vi "GenerateChangedLibrariesList.vi"(6 "GUI Mode? {F)":bool, 8 "error in (no error)":errorcluster) -> (0 "error out":errorcluster)   [LabVIEW 2023, in "CICD.lvlib"]
uses:
  CICD.lvlib
  ead0c1dc-4abe-4fdf-93af-0a2c3e7fff4b.vi
  <vilib>/Wiresmith Technology/G CLI/CLI Class/CLI.lvclass
panel:
  in  "Tab Control":enum32{"GUI Mode", "CLI Mode"}(tab)=enum."CLI Mode"
  in  "Workspace Path":path=path "E:/sw-deps-monitor"
  out "Args":string[](array[string])=["E:\\sw-deps-monitor"]
  # "When in GUI Mode, the controls will be used, \nin CLI Mode the Args will be used"
  # "Command to run the VI from terminal\n\ng-cli -v --lv-ver 2023 --arch 32 \"E:\\sw-deps-monitor\\CICD\\CheckModifiedVIs\\GenerateChangedLibrariesList.vi\" -- \"E:\\sw-deps-monitor\""
  # "Workspace Path"
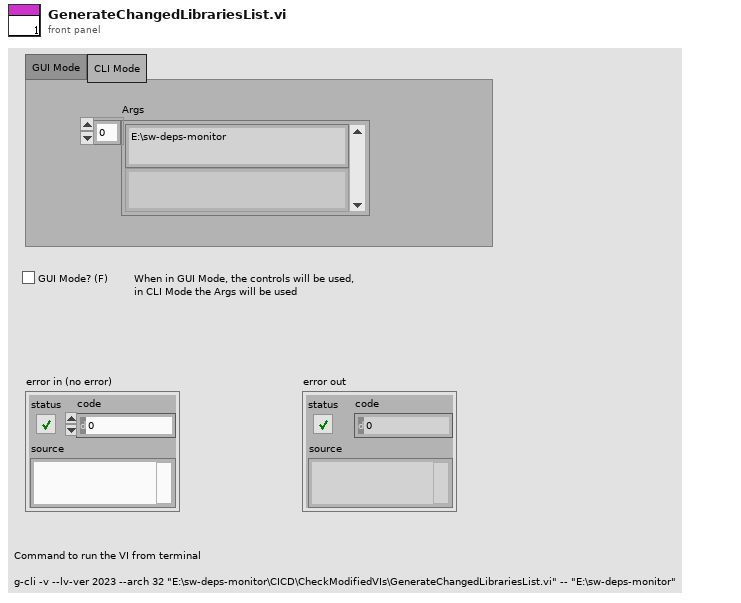
[diagram p1: front panel]
types:
  T1 = enum16{"open", "replace", "create", "open or create", "replace or create", "replace or create with confirmation"}
  T2 = typedef "CICD.lvlib/CICDPathConfigs.ctl" = cluster{"GlobalIncludePaths":path[], "GlobalExcludePaths":path[], "BuildSpecsIncludePaths":path[], "ActualDepsIncludePaths":path[], "WorkspacePath":path, "SourceFolderPaths":path[], "ChangedFilesLogpaths":map{string, path}}
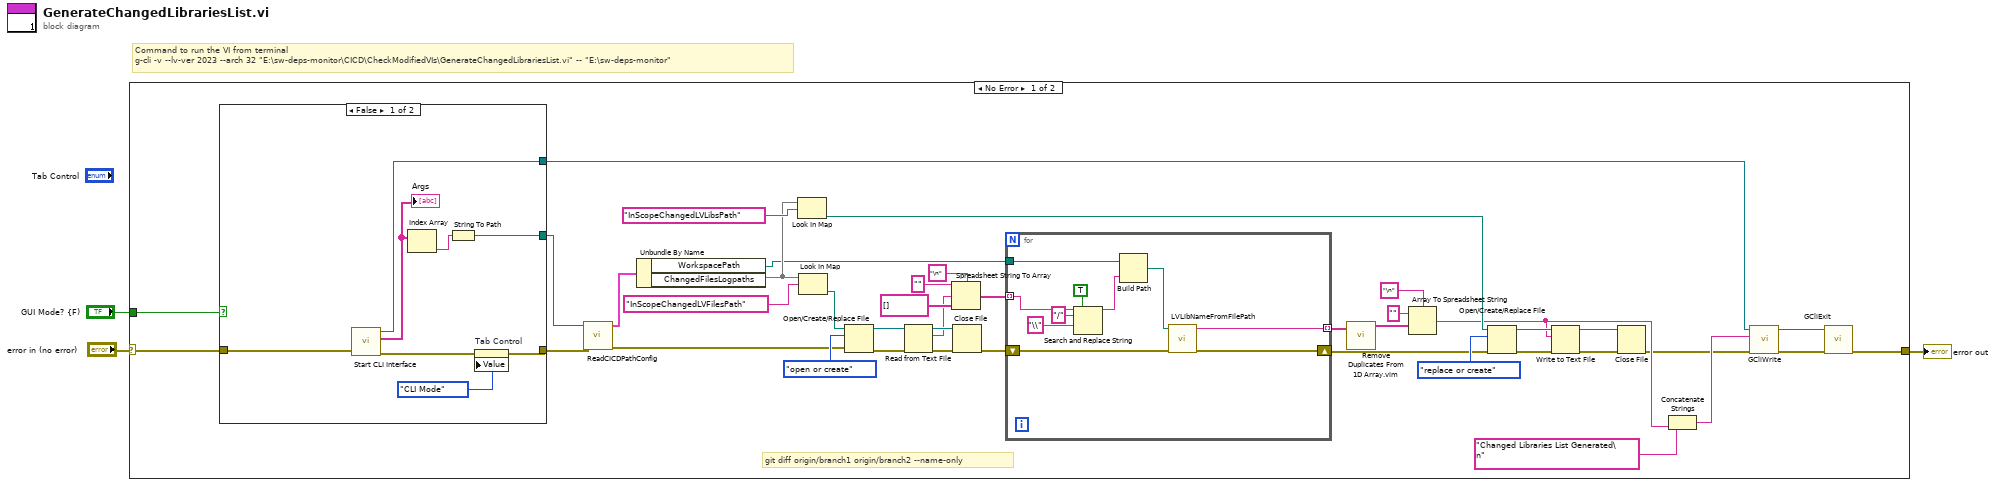
[diagram p0: block diagram]
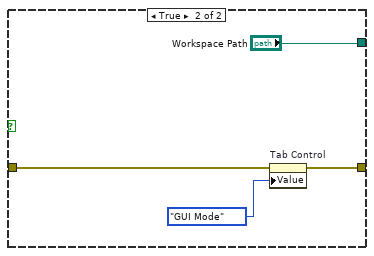
[diagram p2: hidden frame]
diagram:
  # "Command to run the VI from terminal\ng-cli -v --lv-ver 2023 --arch 32 \"E:\\sw-deps-monitor\\CICD\\CheckModifiedVIs\\GenerateChangedLibrariesList.vi\" -- \"E:\\sw-deps-monitor\""
  n1 = case shown="No Error" "error in (no error)" {
    selector: "error in (no error)" -> [w43 w67]
    tunnel: "GUI Mode? {F)" -> [w44 _]
    tunnel: [w39 w67] -> w1
    frame No Error {
      # "git diff origin/branch1 origin/branch2 --name-only"
      n2 = case shown="False" w44 {
        tunnel: [w61 "Workspace Path"] -> w35
        tunnel: w43 -> [w60 w65]
        tunnel: [w58 w63] -> w34
        tunnel: [w59 _] -> w41
        frame False {
          n3 = call <vilib>:"Start CLI Interface.vi"("error in (no error)"=w60) -> ("error out"=w56:errorcluster, "Custom Parameters"=w55:string[], "CLI out"=w59:refnum<class "CLI.lvclass">)  [unwired: 7 in, 1 out]
          "Args" <- w55
          n4 = Index Array(array=w55) -> (element=w62:string)  [unwired: 1 in]
          n5 = String To Path(string=w62) -> (path=w61:path)
          n6 = property on="Tab Control" class="TabCtl (strict)"(error in=w56, "Value"=enum32{"GUI Mode", "CLI Mode"}."CLI Mode" ("Tab Control")) -> (error out=w58:errorcluster)  [unwired: 1 in, 1 out]
        }
        frame True {
          n7 = property on="Tab Control" class="TabCtl (strict)"(error in=w65, "Value"=enum32{"GUI Mode", "CLI Mode"}."GUI Mode" ("Tab Control")) -> (error out=w63:errorcluster)  [unwired: 1 in, 1 out]
        }
      }
      n8 = call "ReadCICDPathConfig.vi"("error in (no error)"=w34, "Workspace Path"=w35) -> ("error out"=w23:errorcluster, "CICD Path Config Out"=w33:T2)  [unwired: 8 in]
      n9 = Unbundle By Name(w33) -> ("WorkspacePath"=w13:path, "ChangedFilesLogpaths"=w21:map{string, path})
      n10 = Look In Map(map=w21, key="InScopeChangedLVLibsPath") -> (value=w20:path)  [unwired: 1 in, 1 out]
      n11 = Look In Map(map=w21, key="InScopeChangedLVFilesPath") -> (value=w31:path)  [unwired: 1 in, 1 out]
      n12 = Open/Create/Replace File(file path (use dialog)=w31, error in=w23, operation (0:open)=T1."open or create") -> (refnum out=w30:refnum<file>, error out=w29:errorcluster)  [unwired: 3 in, 1 out]
      n13 = Read from Text File(file (use dialog)=w30, error in=w29) -> (refnum out=w28:refnum<file>, text=w25:string, error out=w27:errorcluster)  [unwired: 2 in, 1 out]
      n14 = Spreadsheet String To Array(delimiter (Tab)="\n", format string="", spreadsheet string=w25, array type (2D Dbl)=string[] []) -> (array=w14:string[])
      n15 = Close File(refnum=w28, error in=w27) -> (error out=w12:errorcluster)  [unwired: 1 out]
      n16 = for {
        tunnel: w14 -> [w49] mode=indexing
        tunnel: w13 -> [w54]
        tunnel: [w51] -> w5 mode=indexing
        shift-right: [w50] -> w9
        shift-left: w12 -> [w53]
        n17 = Search and Replace String(replace all?=TRUE ("replace all? (F)"), input string=w49, search string="/", replace string="\\" ("replace string (\"\")")) -> (result string=w45:string)  [unwired: 4 in, 3 out]
        n18 = Build Path(base path=w54, name or relative path=w45) -> (appended path=w52:path)
        n19 = call "LVLibNameFromFilePath.vi"("error in (no error)"=w53, "LV File Path"=w52) -> ("error out"=w50:errorcluster, "Library Name"=w51:string)  [unwired: 8 in]
      }
      n20 = call "Remove Duplicates From 1D Array.vim"("array"=w5) -> ("array with duplicates removed"=w4:string[])  [unwired: 10 in]
      n21 = Array To Spreadsheet String(delimiter (Tab)="\n", array=w4, 3:"" ("format string")) -> (spreadsheet string=w8:string)
      n22 = Open/Create/Replace File(file path (use dialog)=w20, error in=w9, operation (0:open)=T1."replace or create") -> (refnum out=w17:refnum<file>, error out=w18:errorcluster)  [unwired: 3 in, 1 out]
      n23 = Write to Text File(file (use dialog)=w17, text=w8, error in=w18) -> (refnum out=w15:refnum<file>, error out=w16:errorcluster)  [unwired: 1 in, 1 out]
      n24 = Close File(refnum=w15, error in=w16) -> (error out=w7:errorcluster)  [unwired: 1 out]
      n25 = Concatenate Strings("Changed Libraries List Generated\n" ("Text to Write"), w8) -> (w36:string)
      n26 = call "GCliWrite.vi"("error in (no error)"=w7, "Text to Write"=w36, "CLI in"=w41) -> ("error out"=w40:errorcluster, "CLI out"=w38:refnum<class "CLI.lvclass">)  [unwired: 7 in]
      n27 = call "GCliExit.vi"("error in (no error)"=w40, "CLI in"=w38) -> ("error out"=w39:errorcluster)  [unwired: 9 in]
    }
    frame Error {
    }
  }
  "error out" <- w1
